vi "Test.ZMQ.vi"() -> ()   [LabVIEW 2014]
panel:
  out "Now (us)":dbl=1.0 format="%.2f"
  in  "Parameter":u16(ring) items=["Frequency (MHz)", "Amplitude (dBm)", "Phase (Pi)"]
  in  "Start":dbl=1.0 format="%.3f"
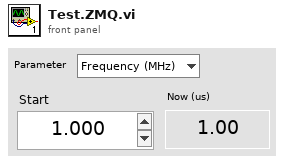
[diagram p1: front panel]
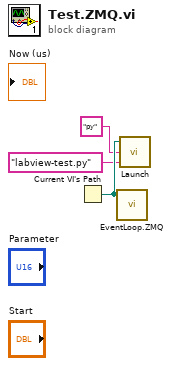
[diagram p0: block diagram]
diagram:
  n1 = Current VI's Path() -> (path=w3:path)
  n2 = call "EventLoop.ZMQ.vi"("Path"=w3) -> ()  [unwired: 2 in]
  n3 = call "Launch.vi"("File"="labview-test.py", "Cmd"="py", "Path"=w3) -> ()
